vi "Async Get averaged image from CamServer and display locally.vi"(4 "Quality":u32=750 max=1000, 6 "Resolution":T1 items=["Low", "Med.", "High", "Max."], 7 "Camera":T3="Travcam", 8 "Averaging time (s) (from end)":dbl=1.0 format="%#_13g", 9 "Duration (s)":dbl=10.0 format="%#_13g", 10 "Image directory path":path=path "C:/test", 11 "Image name":string="test") -> (0 "Error out":errorcluster, 3 "Image file path":path)   [LabVIEW 2015]
doc: "Asynchronously gets a snapshot image from the selected camera on the camera server and saves it to the specified path with specified name. The VI then shows its front panel with the image."
uses:
  Camera enum/Camera enum.ctl
  Camera enum/Camera resolution.ctl
  <vilib>/vision/Image Controls.llb/IMAQ Image.ctl
  Globals/CamServer global.vi
panel:
  out "Image":T2(plugin-control)
  # "PN 21/08/15"
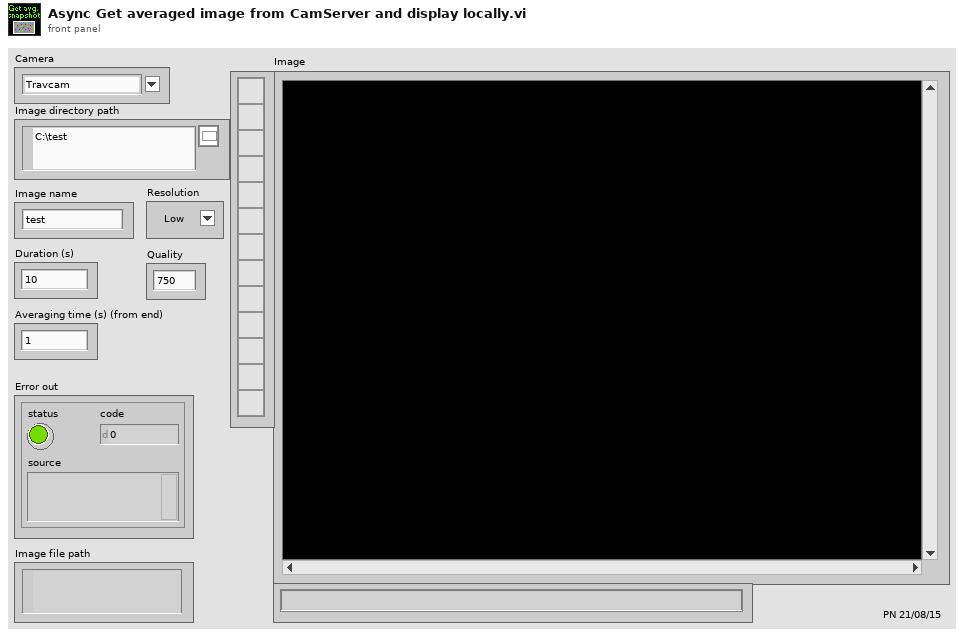
[diagram p1: front panel]
types:
  T1 = typedef "Camera resolution.ctl" = u8
  T2 = typedef "IMAQ Image.ctl" = refnum<image>
  T3 = typedef "Camera enum.ctl" = string
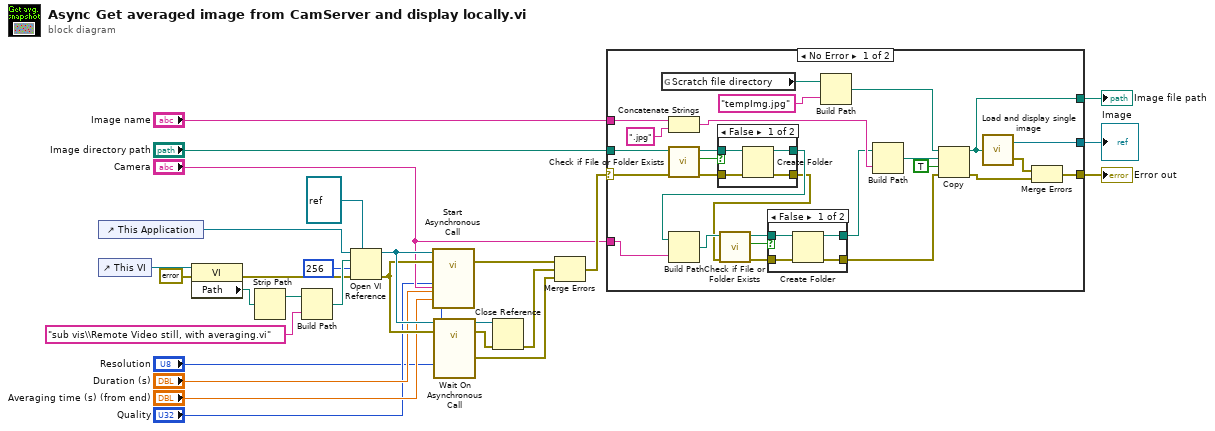
[diagram p0: block diagram]
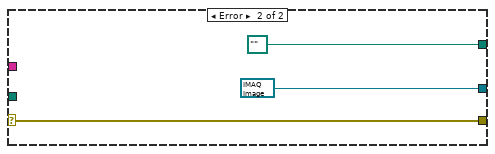
[diagram p4: hidden frame]
diagram:
  n1 = control-ref of="This Application"() -> (w23:refnum<vi>)
  n2 = control-ref of="This VI"() -> (w28:refnum<vi>)
  n3 = property class="VI"(reference=w28, error in=errorcluster {"status"=FALSE, "code"=0, "source"=""} ("error in (no error)")) -> (error out=w25:errorcluster, "Path"=w21:path)  [unwired: 1 out]
  n4 = Strip Path(path=w21) -> (stripped path=w20:path)  [unwired: 1 out]
  n5 = Build Path(base path=w20, name or relative path="sub vis\\Remote Video still, with averaging.vi") -> (appended path=w26:path)
  n6 = Open VI Reference(type specifier VI Refnum (for type only)=refnum<vi> refnum, application reference (local)=w23, vi path=w26, options=256, error in (no error)=w25) -> (vi reference=w19:refnum<vi>, error out=w18:errorcluster)  [unwired: 1 in]
  n7 = call-by-ref "Start Asynchronous Call"(reference=w19, error in=w18, "Resolution"="Resolution", "Quality"="Quality", "Duration (s)"="Duration (s)", "Averaging time (s) (from end)"="Averaging time (s) (from end)", "Camera"="Camera") -> (error out=w16:errorcluster)  [unwired: 2 out]
  n8 = call-by-ref "Wait On Asynchronous Call"(reference=w19, error in=w18) -> (reference out=w17:refnum<vi>, error out=w15:errorcluster, "Error out"=w13:errorcluster)  [unwired: 5 in]
  n9 = Close Reference(reference=w17, error in (no error)=w15) -> (error out=w14:errorcluster)
  n10 = Merge Errors(w16, w14, w13) -> (w12:errorcluster)
  n11 = case shown="No Error" w12 {
    selector: w12 -> [w54 w70]
    tunnel: "Image directory path" -> [w55 _]
    tunnel: "Image name" -> [w49 _]
    tunnel: [w43 w70] -> w9
    tunnel: [w42 T2 refnum ("Image")] -> w8
    tunnel: "Camera" -> [w34 _]
    tunnel: [w29 path "" ("new path")] -> w3
    frame No Error {
      n12 = global read "CamServer global.vi" "Scratch file directory"() -> (w44:path)
      n13 = Concatenate Strings(w49, ".jpg" ("string")) -> (w47:string)
      n14 = call <vilib>:"Check if File or Folder Exists.vi"("error in (no error)"=w54, "path"=w55) -> ("error out"=w51:errorcluster, "file or folder exists?"=w53:bool, "dup path"=w52:path)  [unwired: 7 in]
      n15 = case shown="False" w53 {
        tunnel: w52 -> [w65 w67]
        tunnel: w51 -> [w64 w66]
        tunnel: [w63 w67] -> w35
        tunnel: [w62 w66] -> w32
        frame False {
          n16 = Create Folder(path (use dialog)=w65, error in=w64) -> (created path=w63:path, error out=w62:errorcluster)  [unwired: 1 in, 1 out]
        }
        frame True {
        }
      }
      n17 = Build Path(base path=w35, name or relative path=w34) -> (appended path=w33:path)
      n18 = call <vilib>:"Check if File or Folder Exists.vi"("error in (no error)"=w32, "path"=w33) -> ("error out"=w36:errorcluster, "file or folder exists?"=w37:bool, "dup path"=w38:path)  [unwired: 7 in]
      n19 = case shown="False" w37 {
        tunnel: w38 -> [w59 w61]
        tunnel: w36 -> [w58 w60]
        tunnel: [w57 w61] -> w31
        tunnel: [w56 w60] -> w30
        frame False {
          n20 = Create Folder(path (use dialog)=w59, error in=w58) -> (created path=w57:path, error out=w56:errorcluster)  [unwired: 1 in, 1 out]
        }
        frame True {
        }
      }
      n21 = Build Path(base path=w44, name or relative path="tempImg.jpg") -> (appended path=w40:path)
      n22 = Build Path(base path=w31, name or relative path=w47) -> (appended path=w48:path)
      n23 = Copy(8:w30, 9:TRUE ("overwrite (F)"), 10:w48, 11:w40) -> (0:w41:errorcluster, 3:w29:path)  [unwired: 1 in, 1 out]
      n24 = call "Load and display single image.vi"("Image file path"=w29) -> ("Image"=w42:T2, "Load image error"=w39:errorcluster)
      n25 = Merge Errors(w39, w41) -> (w43:errorcluster)
    }
    frame Error {
    }
  }
  "Error out" <- w9
  "Image" <- w8
  "Image file path" <- w3
